vi "Example.vi"() -> (0 "error out":errorcluster, 3 "ParsedData":T1)   [LabVIEW 2022 SP3, in "ArgumentParser.lvlib"]
uses:
  ArgumentParser.lvlib
  ArgumentParser/_ParsedData.ctl
  ArgumentParser/ArgumentParser.lvclass
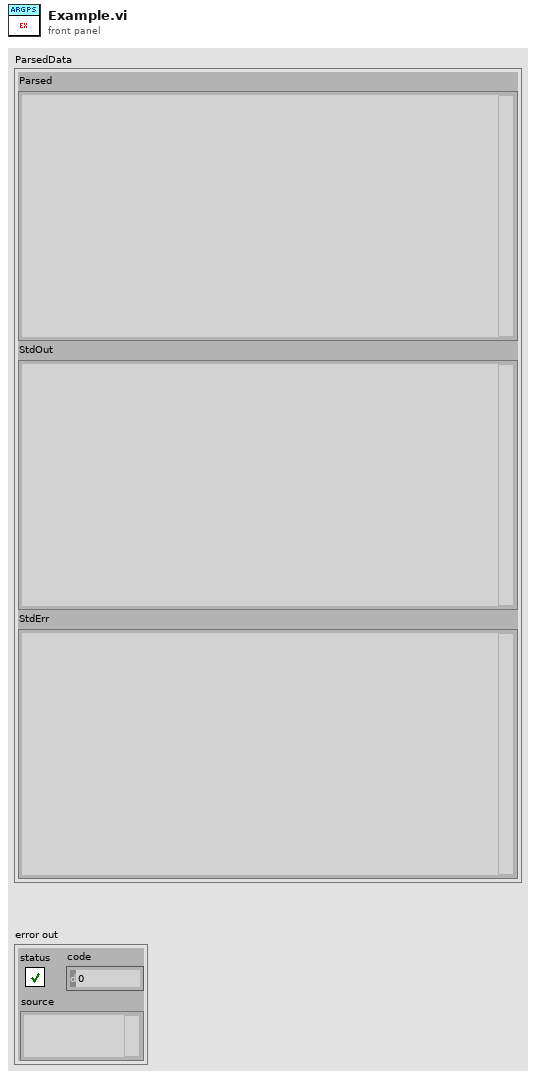
[diagram p1: front panel]
types:
  T1 = typedef "ArgumentParser.lvlib/ArgumentParser.lvclass/_ParsedData.ctl" = cluster{"Parsed":string, "StdOut":string, "StdErr":string}
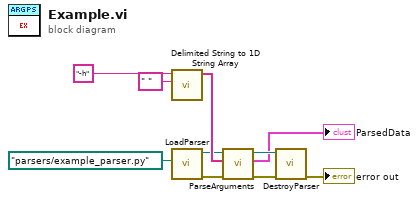
[diagram p0: block diagram]
diagram:
  n1 = call <vilib>:"Delimited String to 1D String Array.vi"("delimiter"=" ", "delimited string"="-h") -> ("string array"=w4:string[])  [unwired: 9 in]
  n2 = call "LoadParser.vi"("ParserPath"=path "parsers/example_parser.py" ("Path")) -> ("error out"=w9:errorcluster, "ArgumentParser"=w2:refnum<class "ArgumentParser.lvclass">)  [unwired: 9 in]
  n3 = call-dynamic "ParseArguments.vi"("error in (no error)"=w9, "CliArguments"=w4, "ArgumentParser in"=w2) -> ("error out"=w8:errorcluster, "ParsedData"=→"ParsedData":T1, "ArgumentParser out"=w7:refnum<class "ArgumentParser.lvclass">)  [unwired: 6 in]
  n4 = call-dynamic "DestroyParser.vi"("error in (no error)"=w8, "ArgumentParser in"=w7) -> ("error out"=→"error out":errorcluster)  [unwired: 9 in]
